vi "ImageQuality.vi"(0 "Quality":u8(slide)=11 scale=1.0..8.0, 2 "SRV In":string) -> (4 "SRV Out":string="169.254.0.10")   [LabVIEW 2009]
panel:
  out "Reply":string
  # "1 is high and 8 is low"
  # "This LabVIEW item is deprecated.\n\nIt is believed to be unused and will be removed in a future version of SRV."
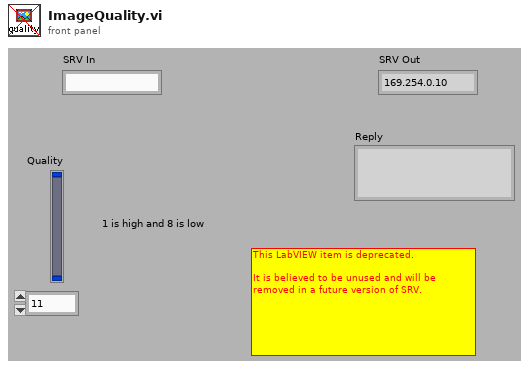
[diagram p1: front panel]
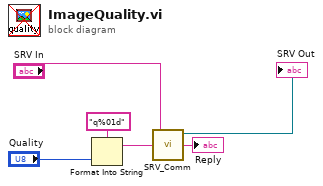
[diagram p0: block diagram]
diagram:
  n1 = Format Into String(format string="q%01d" ("Command Sent"), "Quality") -> (resulting string=w4:string)  [unwired: 2 in, 1 out]
  n2 = call "SRV_Comm.vi"("Command Sent"=w4, "SRV In"="SRV In") -> ("Reply"=→"Reply":string, "SRV Out"=→"SRV Out":refnum<k5>)  [unwired: 1 in, 1 out]
